vi "Set Device.vi"(8 "error in (no error)":errorcluster, 9 "Length":i32=1, 10 "Head Address":string="000", 11 "Device Type":string="D") -> (0 "error out":errorcluster, 3 "Device":refnum<class "Device.lvclass">)   [LabVIEW 2019, in "SLMP.lvlib" / "Device.lvclass"]
uses:
  Device.lvclass
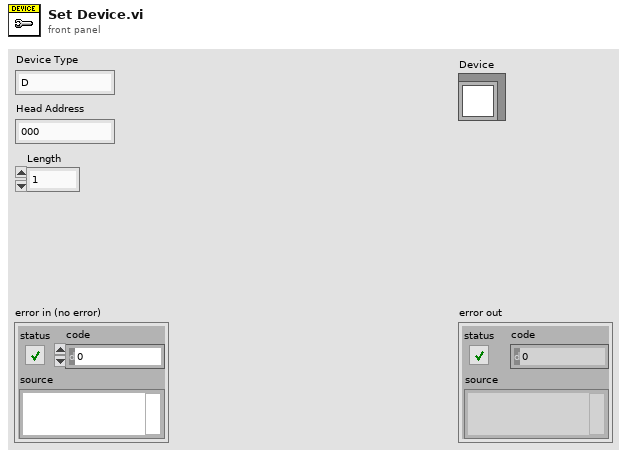
[diagram p1: front panel]
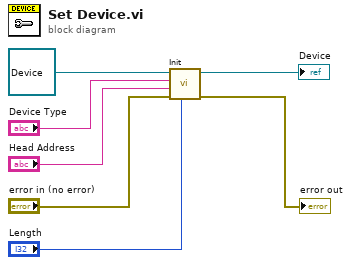
[diagram p0: block diagram]
diagram:
  n1 = call "Init.vi"("Number of devices"="Length", "error in (no error)"="error in (no error)", "Head Device No"="Head Address", "Device Type"="Device Type", "Device in"=refnum<class "Device.lvclass"> refnum ("SLMP.lvlib:Device.lvclass")) -> ("error out"=→"error out":errorcluster, "Device out"=→"Device":refnum<class "Device.lvclass">)  [unwired: 5 in]
